vi "Initialize.vi"(8 "error in (no error)":errorcluster, 11 "View Template in":refnum<class "[M] TDMS Save.lvclass">) -> (0 "error out":errorcluster, 3 "View Template out":refnum<class "[M] TDMS Save.lvclass">)   [LabVIEW 2020, in "[M] TDMS Save.lvlib" / "[M] TDMS Save.lvclass"]
uses:
  [M] TDMS Save.lvclass
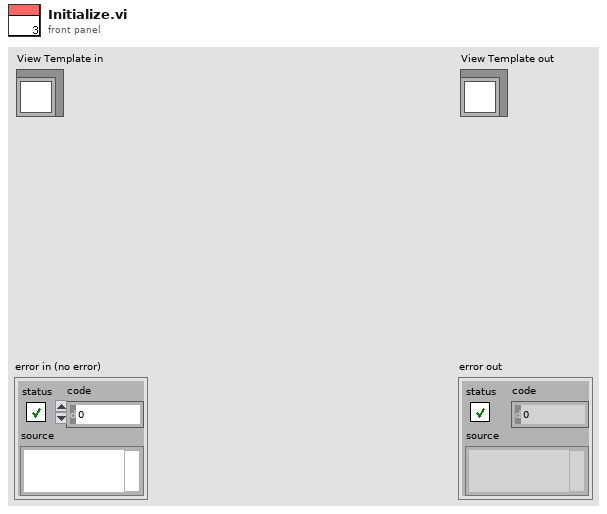
[diagram p1: front panel]
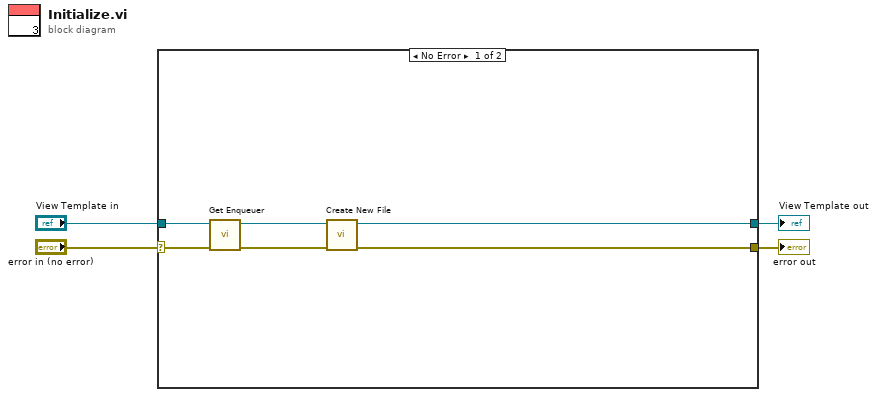
[diagram p0: block diagram]
diagram:
  n1 = case shown="No Error" "error in (no error)" {
    selector: "error in (no error)" -> [w9 w12]
    tunnel: [w7 w12] -> w3
    tunnel: [w5 w11] -> w1
    tunnel: "View Template in" -> [w10 w11]
    frame No Error {
      n2 = call "Get Enqueuer.vi"("error in (no error)"=w9, "View Template in"=w10) -> ("error out"=w8:errorcluster, "View Template out"=w6:refnum<class "[M] TDMS Save.lvclass">)  [unwired: 8 in]
      n3 = call "Create New File.vi"("error in (no error)"=w8, "[M] TDMS Save in"=w6) -> ("error out"=w7:errorcluster, "[M] TDMS Save out"=w5:refnum<class "[M] TDMS Save.lvclass">)  [unwired: 8 in]
    }
    frame Error {
    }
  }
  "error out" <- w3
  "View Template out" <- w1
